vi "dw.vi"(0 "Port":i32, 1 "String 2":string, 2 "Delay(ms)":u32=10, 3 "error in (no error)":errorcluster) -> (4 "# of Bytes Read":u32=50, 5 "String Read 2":string, 6 "String":string, 7 "error out":errorcluster, 8 "error out 2":errorcluster)   [LabVIEW 2017]
panel:
  in  "VISA resource name out":refnum<visa-resource-name>
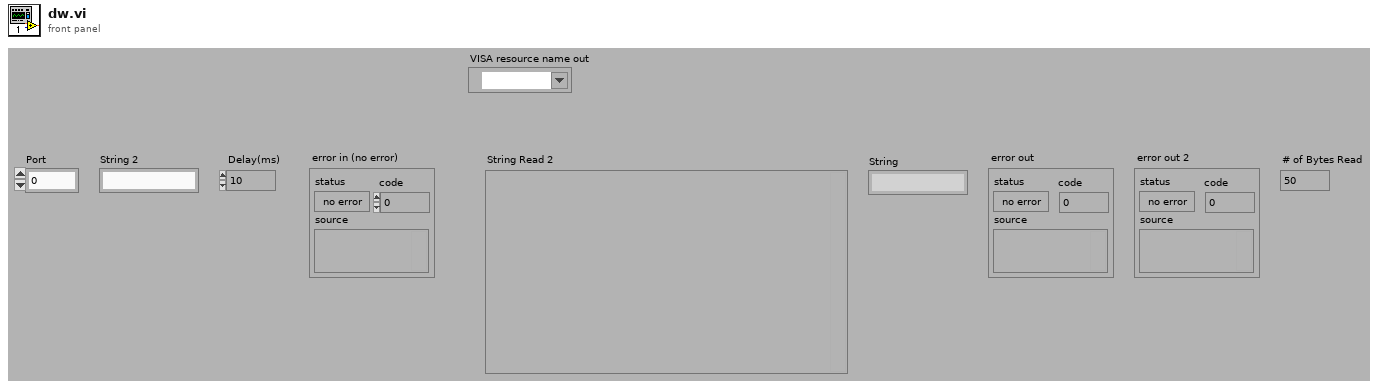
[diagram p1: front panel]
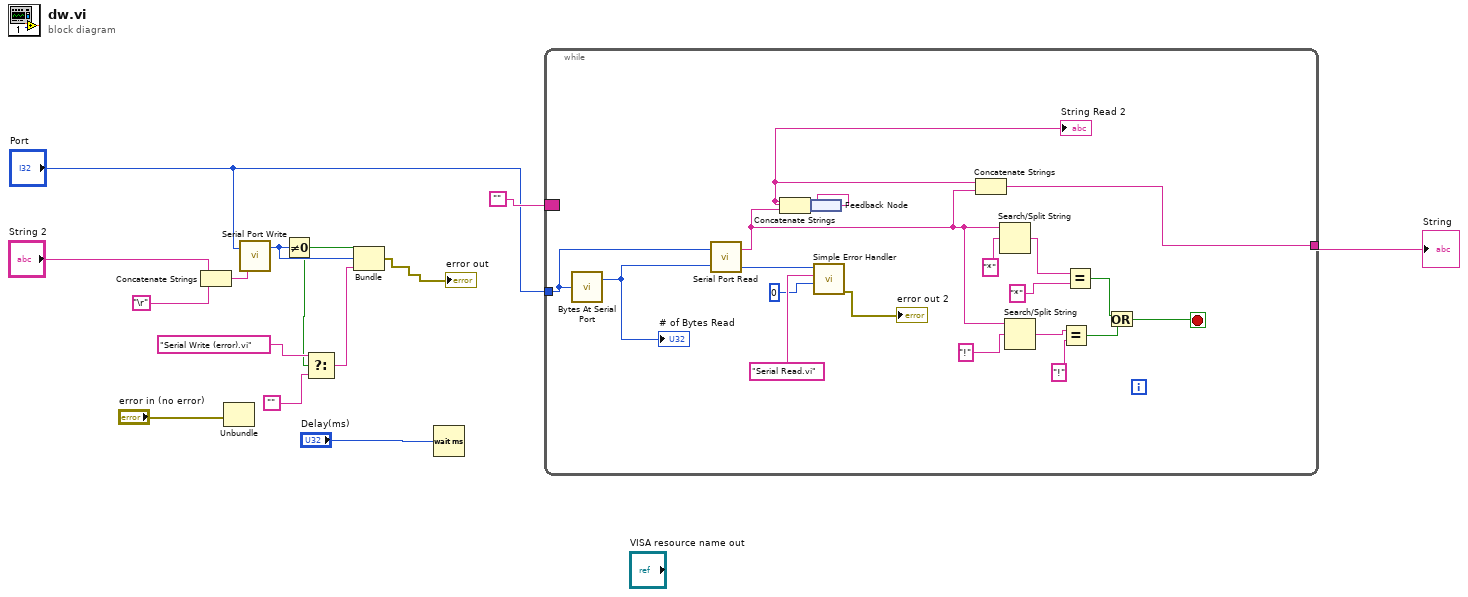
[diagram p0: block diagram]
diagram:
  n1 = Concatenate Strings("String 2", "\r") -> (w8:string)
  n2 = Unbundle("error in (no error)") -> ()  [unwired: 3 out]
  n3 = call <vilib>:"Serial Port Write.vi"("string to write"=w8, "port number"="Port") -> ("error code"=w9:i32)
  n4 = Not Equal To 0?(x=w9) -> (x != 0?=w2:bool)
  n5 = Select(t="Serial Write (error).vi", s=w2, f="") -> (s? t:f=w1:string)
  n6 = Bundle(w2, "error code"=w9, w1) -> (→"error out":cluster{bool, "error code":i32, string})  [unwired: 1 in]
  n7 = Wait (ms)(milliseconds to wait="Delay(ms)") -> ()  [unwired: 1 out]
  n8 = while {
    tunnel: "Port" -> [w29]
    tunnel: [w24] -> w13
    border: "" -> [_]
    stop <- w15 stop-if-true
    n9 = call <vilib>:"Bytes At Serial Port.vi"("port number"=w29) -> ("byte count"=w30:u32)  [unwired: 1 out]
    "# of Bytes Read" <- w30
    n10 = call <vilib>:"Serial Port Read.vi"("requested byte count"=w30, "port number"=w29) -> ("error code"=w33:i32, "string read"=w22:string)
    n11 = feedback #1() -> (w16:string)
    "String Read 2" <- w16
    n12 = Concatenate Strings(w16, w22) -> (w26:string)
    n13 = feedback-in #1(w26) -> ()
    n14 = call <vilib>:"Simple Error Handler.vi"("error code (no error:0)"=w33, "error source (\" \")"="Serial Read.vi", "type of dialog (OK msg:1)"=0) -> ("error out"=→"error out 2":errorcluster)  [unwired: 2 in, 4 out]
    n15 = Concatenate Strings(w16, w22) -> (w24:string)
    n16 = Search/Split String(string=w22, search string/char (-)="*") -> (match + rest of string=w25:string)  [unwired: 1 in, 2 out]
    n17 = Search/Split String(string=w22, search string/char (-)="!") -> (match + rest of string=w20:string)  [unwired: 1 in, 2 out]
    n18 = Equal?(x=w20, y="!") -> (x = y?=w17:bool)
    n19 = Equal?(x=w25, y="*") -> (x = y?=w18:bool)
    n20 = Or(x=w18, y=w17) -> (x .or. y?=w15:bool)
  }
  "String" <- w13
